vi "Init Main Page Connections GUI.vi"(5 "Mode Desciption":refnum<vi>, 7 "Controls":refnum<vi>[](array[refnum]), 8 "error in (no error)":errorcluster, 11 "AutoSelection":T1={"Mode"=enum."Generate sample clock", "pxitrig"=FALSE, "pfi0"=TRUE, "pfi1"=TRUE, "pfi2"=TRUE, "External Pin"=enum."PFI0", "Routes"=[]}) -> (0 "error out":errorcluster)   [LabVIEW 2011, in "Chassis TimeSync System Explorer.lvlib"]
uses:
  Chassis TimeSync System Explorer.lvlib
  Shared/Connection Settings.ctl
  Shared/Mode.ctl
  Shared/External Pin.ctl
  Shared/Routes.ctl
  Shared/Route.ctl
  sub_EnableDisable Control.vi
  Shared/Chassis TimeSync Shared.lvlib
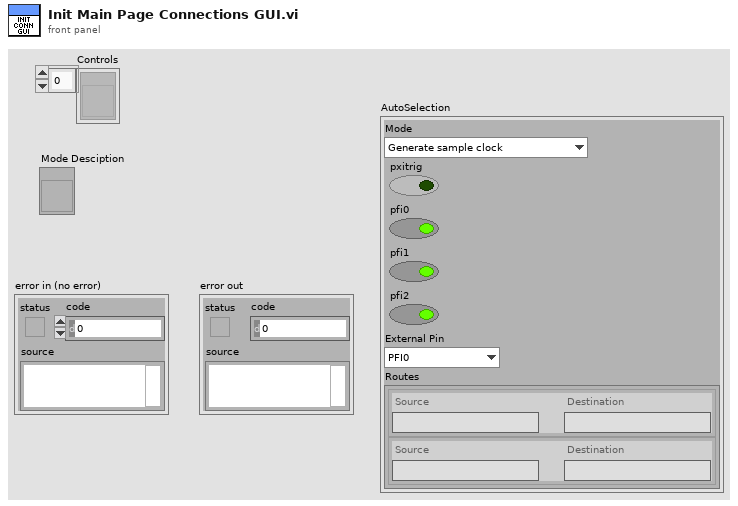
[diagram p1: front panel]
types:
  T1 = typedef "Chassis TimeSync Shared.lvlib/Connection Settings.ctl" = cluster{"Mode":T2, "pxitrig":bool, "pfi0":bool, "pfi1":bool, "pfi2":bool, "External Pin":T3, "Routes":T4}
  T2 = typedef "Chassis TimeSync Shared.lvlib/Mode.ctl" = enum16{"Generate sample clock", "Route sample clock out of chassis", "Route sample clock into chassis", "Custom routes"}
  T3 = typedef "Chassis TimeSync Shared.lvlib/External Pin.ctl" = enum16{"PFI0", "PFI1", "PFI2"}
  T4 = typedef "Chassis TimeSync Shared.lvlib/Routes.ctl" = T5[]
  T5 = typedef "Chassis TimeSync Shared.lvlib/Route.ctl" = cluster{"Source":string, "Destination":string}
  T6 = typedef "Chassis TimeSync System Explorer.lvlib/Pins Tab.ctl" = enum32{"Pins", "Ext. Pin", "Custom"}
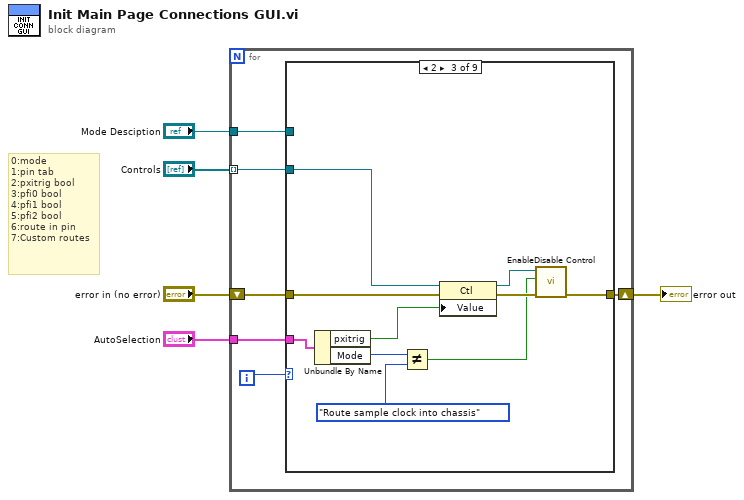
[diagram p0: block diagram]
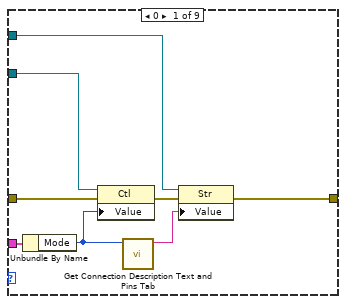
[diagram p2: hidden frame]
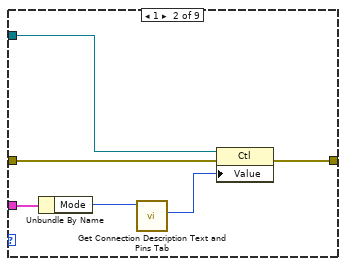
[diagram p3: hidden frame]
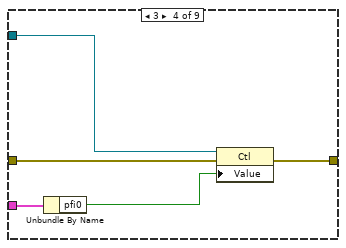
[diagram p4: hidden frame]
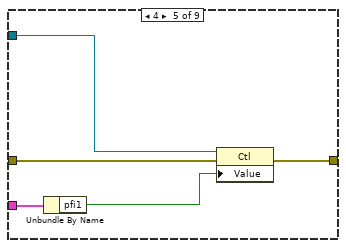
[diagram p5: hidden frame]
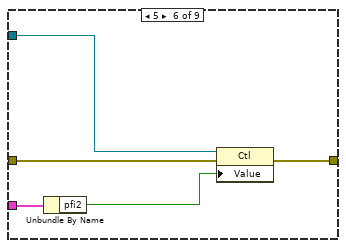
[diagram p6: hidden frame]
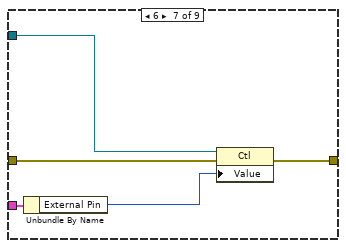
[diagram p7: hidden frame]
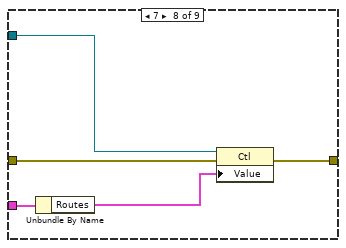
[diagram p8: hidden frame]
diagram:
  # "0:mode\n1:pin tab\n2:pxitrig bool\n3:pfi0 bool\n4:pfi1 bool\n5:pfi2 bool\n6:route in pin\n7:Custom routes"
  n1 = for {
    shift-right: [w7] -> w3
    shift-left: "error in (no error)" -> [w9]
    tunnel: "Controls" -> [w8] mode=indexing
    tunnel: "AutoSelection" -> [w11]
    tunnel: "Mode Desciption" -> [w6]
    i -> [w10]
    n2 = case shown="2" w10 {
      tunnel: w11 -> [w19 w25 w35 w40 w45 w50 w55 w60 _]
      tunnel: w9 -> [w18 w24 w34 w39 w44 w49 w54 w59 w61]
      tunnel: w8 -> [w17 w23 w33 w38 w43 w48 w53 w58 _]
      tunnel: [w12 w22 w30 w36 w41 w46 w51 w56 w61] -> w7
      tunnel: w6 -> [w15 _ _ _ _ _ _ _ _]
      frame 0 {
        n3 = Unbundle By Name(w19) -> ("Mode"=w14:T2)
        n4 = property class="Ctl"(reference=w17, error in=w18, "Value"=w14) -> (error out=w16:errorcluster)  [unwired: 1 out]
        n5 = call "Get Connection Description Text and Pins Tab.vi"("Mode"=w14) -> ("Description"=w13:string)  [unwired: 9 in, 1 out]
        n6 = property class="Str"(reference=w15, error in=w16, "Value"=w13) -> (error out=w12:errorcluster)  [unwired: 1 out]
      }
      frame 1 {
        n7 = Unbundle By Name(w25) -> ("Mode"=w21:T2)
        n8 = call "Get Connection Description Text and Pins Tab.vi"("Mode"=w21) -> ("Pins tab"=w20:T6)  [unwired: 9 in, 1 out]
        n9 = property class="Ctl"(reference=w23, error in=w24, "Value"=w20) -> (error out=w22:errorcluster)  [unwired: 1 out]
      }
      frame 2 {
        n10 = Unbundle By Name(w35) -> ("pxitrig"=w32:bool, "Mode"=w28:T2)
        n11 = Not Equal?(x=w28, y=Mode."Route sample clock into chassis") -> (x != y?=w26:bool)
        n12 = property class="Ctl"(reference=w33, error in=w34, "Value"=w32) -> (reference out=w29:refnum<vi>, error out=w31:errorcluster)
        n13 = call-poly "EnableDisable Control.vi"("error in (no error)"=w31, "Enable"=w26, "Control"=w29) -> ("error out"=w30:errorcluster)  [unwired: 8 in]
      }
      frame 3 {
        n14 = Unbundle By Name(w40) -> ("pfi0"=w37:bool)
        n15 = property class="Ctl"(reference=w38, error in=w39, "Value"=w37) -> (error out=w36:errorcluster)  [unwired: 1 out]
      }
      frame 4 {
        n16 = Unbundle By Name(w45) -> ("pfi1"=w42:bool)
        n17 = property class="Ctl"(reference=w43, error in=w44, "Value"=w42) -> (error out=w41:errorcluster)  [unwired: 1 out]
      }
      frame 5 {
        n18 = Unbundle By Name(w50) -> ("pfi2"=w47:bool)
        n19 = property class="Ctl"(reference=w48, error in=w49, "Value"=w47) -> (error out=w46:errorcluster)  [unwired: 1 out]
      }
      frame 6 {
        n20 = Unbundle By Name(w55) -> ("External Pin"=w52:T3)
        n21 = property class="Ctl"(reference=w53, error in=w54, "Value"=w52) -> (error out=w51:errorcluster)  [unwired: 1 out]
      }
      frame 7 {
        n22 = Unbundle By Name(w60) -> ("Routes"=w57:T4)
        n23 = property class="Ctl"(reference=w58, error in=w59, "Value"=w57) -> (error out=w56:errorcluster)  [unwired: 1 out]
      }
      frame Default {
      }
    }
  }
  "error out" <- w3
